vi "Start acquisition.vi"(5 "y frame size":u16, 7 "x frame size":u16, 8 "error in (no error)":errorcluster, 9 "Trigger mode":T1 items=["Timed", "Strobed", "Bulb", "Trigger first"], 10 "Exposure":u32, 11 "camera handle in":i16) -> (0 "error out":errorcluster, 2 "buffer ref out":i32, 3 "camera handle out":i16)   [LabVIEW 2012]
uses:
  Trigger mode.ctl
  Buffer mode.ctl
  Visual Studio/Cascade wrapper/Release/Cascade wrapper.dll
panel:
  out "dimension":i32
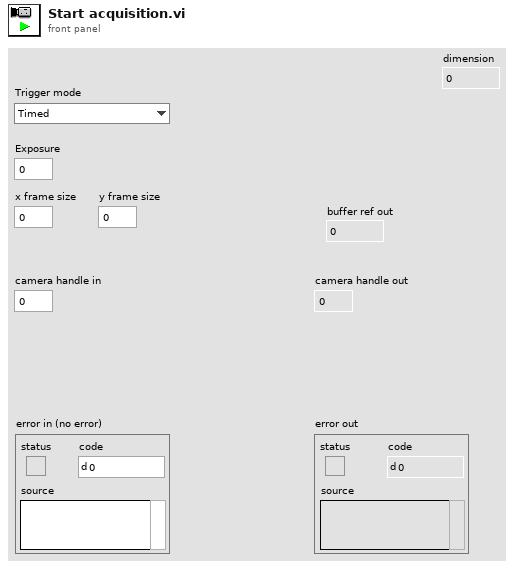
[diagram p1: front panel]
types:
  T1 = typedef "Trigger mode.ctl" = i16
  T2 = typedef "Buffer mode.ctl" = i16
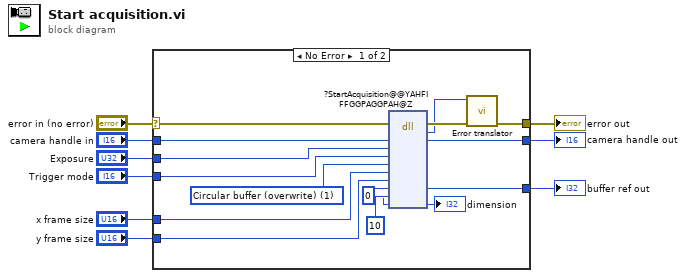
[diagram p0: block diagram]
diagram:
  n1 = case shown="No Error" "error in (no error)" {
    selector: "error in (no error)" -> [w24 w26]
    tunnel: [w21 w26] -> w8
    tunnel: "camera handle in" -> [w20 w25]
    tunnel: [w19 w25] -> w6
    tunnel: "Exposure" -> [w18 _]
    tunnel: "x frame size" -> [w17 _]
    tunnel: "y frame size" -> [w16 _]
    tunnel: [w15 _] -> w2
    tunnel: "Trigger mode" -> [w13 _]
    frame No Error {
      w14 = T2 1 items=["No circular buffer", "Circular buffer (overwrite)", "Circular buffer (no overwrite)"] ("Buffer mode")
      w11 = 0 ("buffer ref")
      n2 = dll-call lib="C:/moroder/Cascade wrapper/Visual Studio/Cascade wrapper/Release/Cascade wrapper.dll" fn="?StartAcquisition@@YAHFIFFGGPAGGPAH@Z"(error in=w24, "camera handle"=w20, "exposure"=w18, "exposure mode"=w13, "circular buffer mode"=w14, "frame x size"=w17, "frame y size"=w16, "buffer ref"=w11, "# frames in buffer"=u16 10 ("# of frames in buffer"), "dimension"=w11) -> (error out=w23:errorcluster, "error"=w22:i32, "camera handle"=w19:i16, "buffer ref"=w15:i32, "dimension"=→"dimension":i32)  [unwired: 8 in, 1 out]
      n3 = call "Error translator.vi"("error in (no error)"=w23, "error code"=w22) -> ("error out"=w21:errorcluster)  [unwired: 9 in]
    }
    frame Error {
    }
  }
  "error out" <- w8
  "camera handle out" <- w6
  "buffer ref out" <- w2
